vi "testRegTel.vi"(8 "error in (no error)":errorcluster) -> (0 "error out":errorcluster)   [LabVIEW 2018]
doc: "Test the regTel.vi."
uses:
  src/TcpServer/TcpServer.lvclass
  src/TcpServer/TcpServer.lvclass/TcpServer.ctl
  src/TcpServerBase/TcpServerBase.lvclass/TcpServerBase.ctl
  src/TcpServerTel/TcpServerTel.lvclass
  home/pcortes/github/ts_labview_tcp_json/src/TcpServerBase/TcpServerBase.lvclass
  <vilib>/addons/_JKI Toolkits/Caraya/classes/Assert/Assert Equal Value_Variant.vi
  <vilib>/addons/_JKI Toolkits/Caraya/classes/Test/Test.lvclass
  <vilib>/addons/_JKI Toolkits/Caraya/classes/Assert/Assert.lvclass
  src/TcpServerBase/TcpServerBase.lvclass
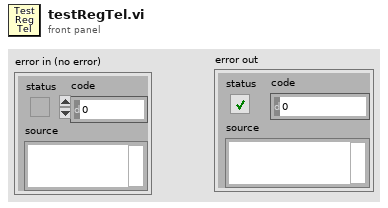
[diagram p1: front panel]
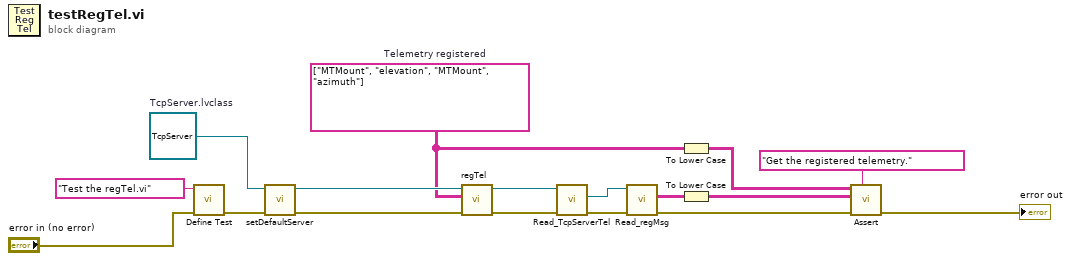
[diagram p0: block diagram]
diagram:
  w7 = string[][] [["MTMount", "elevation"], ["MTMount", "azimuth"]]  # Telemetry registered
  w14 = refnum<class "TcpServer.lvclass"> refnum  # TcpServer.lvclass
  n1 = call <vilib>:"Define Test.vi"("error in (no error)"="error in (no error)", "Label (VI Title)"="Test the regTel.vi") -> ("error out"=w16:errorcluster)  [unwired: 9 in]
  n2 = call "setDefaultServer.vi"("error in (no error)"=w16, "TcpServer.lvclass"=w14) -> ("error out"=w11:errorcluster, "tcpServer out"=w12:refnum<class "TcpServer.lvclass">)  [unwired: 8 in]
  n3 = call "regTel.vi"("error in (no error)"=w11, "telReg"=w7, "tcpServer in"=w12) -> ("error out"=w3:errorcluster, "tcpServer out"=w4:refnum<class "TcpServer.lvclass">)  [unwired: 7 in]
  n4 = call "Read_TcpServerTel.vi"("error in (no error)"=w3, "TcpServer in"=w4) -> ("error out"=w1:errorcluster, "TcpServerTel.lvclass"=w2:refnum<class "TcpServerTel.lvclass">)  [unwired: 7 in, 1 out]
  n5 = call "Read_regMsg.vi"("error in (no error)"=w1, "TcpServerBase in"=w2) -> ("error out"=w9:errorcluster, "regMsg"=w8:string[][])  [unwired: 7 in, 1 out]
  n6 = To Lower Case(string=w7) -> (all lower case string=w5:string[][])
  n7 = To Lower Case(string=w8) -> (all lower case string=w6:string[][])
  n8 = call-poly <vilib>:"Assert.vi"("Label"="Get the registered telemetry.", "error in (no error)"=w9, "Y"=w6, "X"=w5) -> ("error out"=→"error out":errorcluster)  [unwired: 7 in]
